vi "SelectFromArray.vi"(11 "Array in":T1(array[cluster])) -> (3 "Array out":T1(array[cluster]))   [LabVIEW 2014, in "Manipulator.lvclass"]
uses:
  Manipulator.lvclass
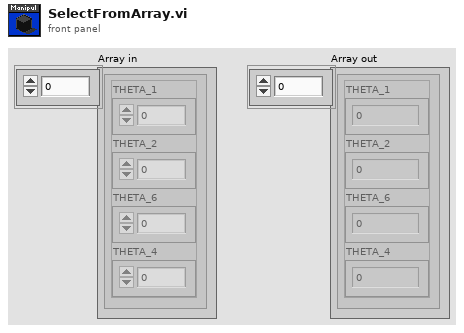
[diagram p1: front panel]
types:
  T1 = cluster{"THETA_1":dbl, "THETA_2":dbl, "THETA_6":dbl, "THETA_4":dbl}[]
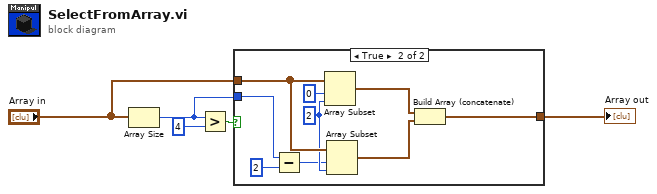
[diagram p0: block diagram]
diagram:
  n1 = Array Size(array="Array in") -> (size(s)=w4:i32)
  n2 = Greater?(x=w4, y=4) -> (0:w3:bool)
  n3 = case shown="True" w3 {
    tunnel: "Array in" -> [w6 w14]
    tunnel: w4 -> [_ w12]
    tunnel: [w6 w7] -> w5
    frame False {
    }
    frame True {
      w13 = 2 ("length")
      n4 = Subtract(x=w12, y=2) -> (x-y=w10:i32)
      n5 = Array Subset(array=w14, index=0, length=w13) -> (w9:T1)
      n6 = Array Subset(array=w14, index=w10, length=w13) -> (w8:T1)
      n7 = Build Array (concatenate)(w9, w8) -> (w7:T1)
    }
  }
  "Array out" <- w5
